vi "Remove_Duplicates_1D.vi"(10 "Input Array":dbl[](array[numeric])) -> (1 "Unique Array":dbl[](array[numeric]), 3 "Removed indicies":i32[](array[numeric]))   [LabVIEW 2012]
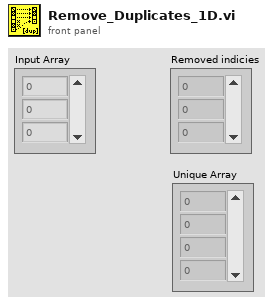
[diagram p1: front panel]
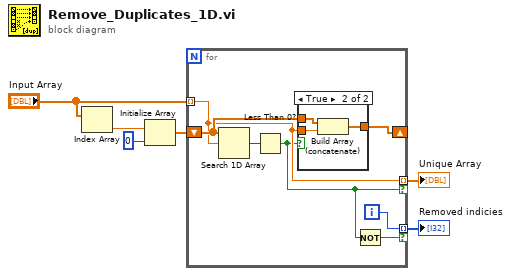
[diagram p0: block diagram]
diagram:
  n1 = Index Array(array="Input Array") -> (element=w4:dbl)  [unwired: 1 in]
  n2 = Initialize Array(w4, 0 ("Dimension Size")) -> (w5:dbl[])
  n3 = for {
    tunnel: "Input Array" -> [w10] mode=indexing
    shift-right: [w13] -> _
    shift-left: w5 -> [w12]
    tunnel: [w10] -> w1 mode=indexing if=w7
    tunnel: [w9] -> w2 mode=indexing if=w8
    i -> [w9]
    n4 = Search 1D Array(1D array=w12, element=w10) -> (index of element=w11:i32)  [unwired: 1 in]
    n5 = Less Than 0?(x=w11) -> (x < 0?=w7:bool)
    n6 = case shown="True" w7 {
      tunnel: w10 -> [_ w17]
      tunnel: [w14 w15] -> w13
      tunnel: w12 -> [w14 w16]
      frame False {
      }
      frame True {
        n7 = Build Array (concatenate)(w16, w17) -> (w15:dbl[])
      }
    }
    n8 = Not(x=w7) -> (.not. x?=w8:bool)
  }
  "Removed indicies" <- w2
  "Unique Array" <- w1
